vi "Generate Pin Map Client.vi"() -> ()   [LabVIEW 2020]
panel:
  out "error out":errorcluster
  in  "error in (no error)":errorcluster
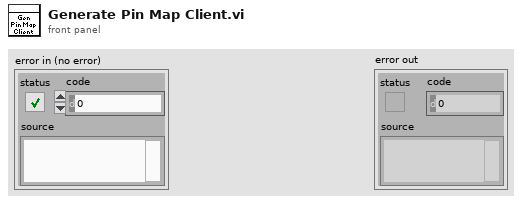
[diagram p1: front panel]
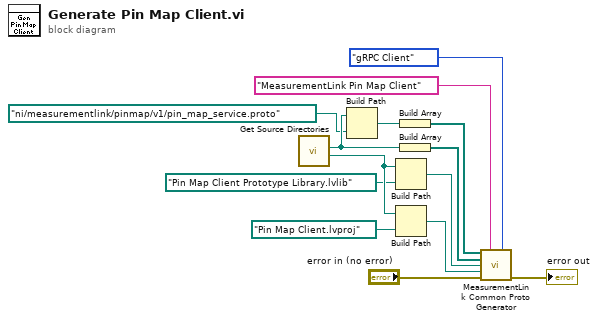
[diagram p0: block diagram]
diagram:
  n1 = call "Get Source Directories.vi"() -> ("Runtime Dir"=w8:path, "Protos Dir"=w4:path)  [unwired: 9 in, 1 out]
  n2 = Build Path(base path=w4, name or relative path=path "ni/measurementlink/pinmap/v1/pin_map_service.proto" ("Proto File Path")) -> (appended path=w5:path)
  n3 = Build Path(base path=w8, name or relative path=path "Pin Map Client Prototype Library.lvlib") -> (appended path=w6:path)
  n4 = Build Path(base path=w8, name or relative path=path "Pin Map Client.lvproj" ("Target Project")) -> (appended path=w9:path)
  n5 = Build Array(w5) -> (w11:path[])
  n6 = Build Array(w4) -> (w12:path[])
  n7 = call "MeasurementLink Common Proto Generator.vi"("Proto File Path"=w11, "Generated Library Full Name"="MeasurementLink Pin Map Client" ("Generated Library Name"), "Generate"=enum16{"gRPC Server", "gRPC Client", "Both"}."gRPC Client", "Import Paths"=w12, "Prototype Library"=w6, "Target Project"=w9, "error in (no error)"="error in (no error)") -> ("error out"=→"error out":errorcluster)  [unwired: 8 in]
